vi "Load Waveform From TDMS.vi"(0 "TDMS File Path":path, 5 "Waveform Name (File Name)":string, 11 "error in (no error)":errorcluster) -> (4 "Waveform":T1={"Waveform Name"="Wfm", "Waveform"={"x0"=0.0, "dx"=0.0, "y"=[]}, "Signal Bandwidth (Hz)"=0.0, "PAPR (dB)"=0.0, "Burst Length (s)"=0.0, "Sample Rate"=0.0, "Burst Start Locations"=[], "Burst Stop Locations"=[], "Idle Duration Present?"=FALSE, "Runtime Scaling"=0.0} {"Runtime Scaling" format="%#_6p"; "Sample Rate" format="%#_6p"; "Burst Length (s)" format="%#_6p"; "PAPR (dB)" format="%.2f"; "Signal Bandwidth (Hz)" format="%.2f"; "Waveform"."y" format="%.2f"; "Waveform"."dx" format="%^.2e"; "Waveform"."x0" format="%^.2e"}, 15 "error out":errorcluster)   [LabVIEW 2016, in "SG.lvlib"]
uses:
  SG.lvlib
  Typedefs/Waveform.ctl
  <instrlib>/niRFSGPlayback/niRFSGPlayback Read Waveform From File (1 Wfm,TDMS, CSG).vi
  Utilities/RDLUtilities.lvlib
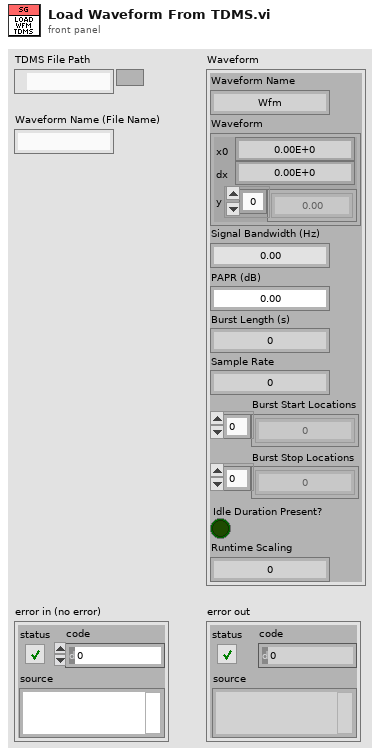
[diagram p1: front panel]
types:
  T1 = typedef "SG.lvlib/Waveform.ctl" = cluster{"Waveform Name":string, "Waveform":cluster{"x0":dbl, "dx":dbl, "y":csg[]}, "Signal Bandwidth (Hz)":dbl, "PAPR (dB)":dbl, "Burst Length (s)":dbl, "Sample Rate":dbl, "Burst Start Locations":i32[], "Burst Stop Locations":i32[], "Idle Duration Present?":bool, "Runtime Scaling":dbl}
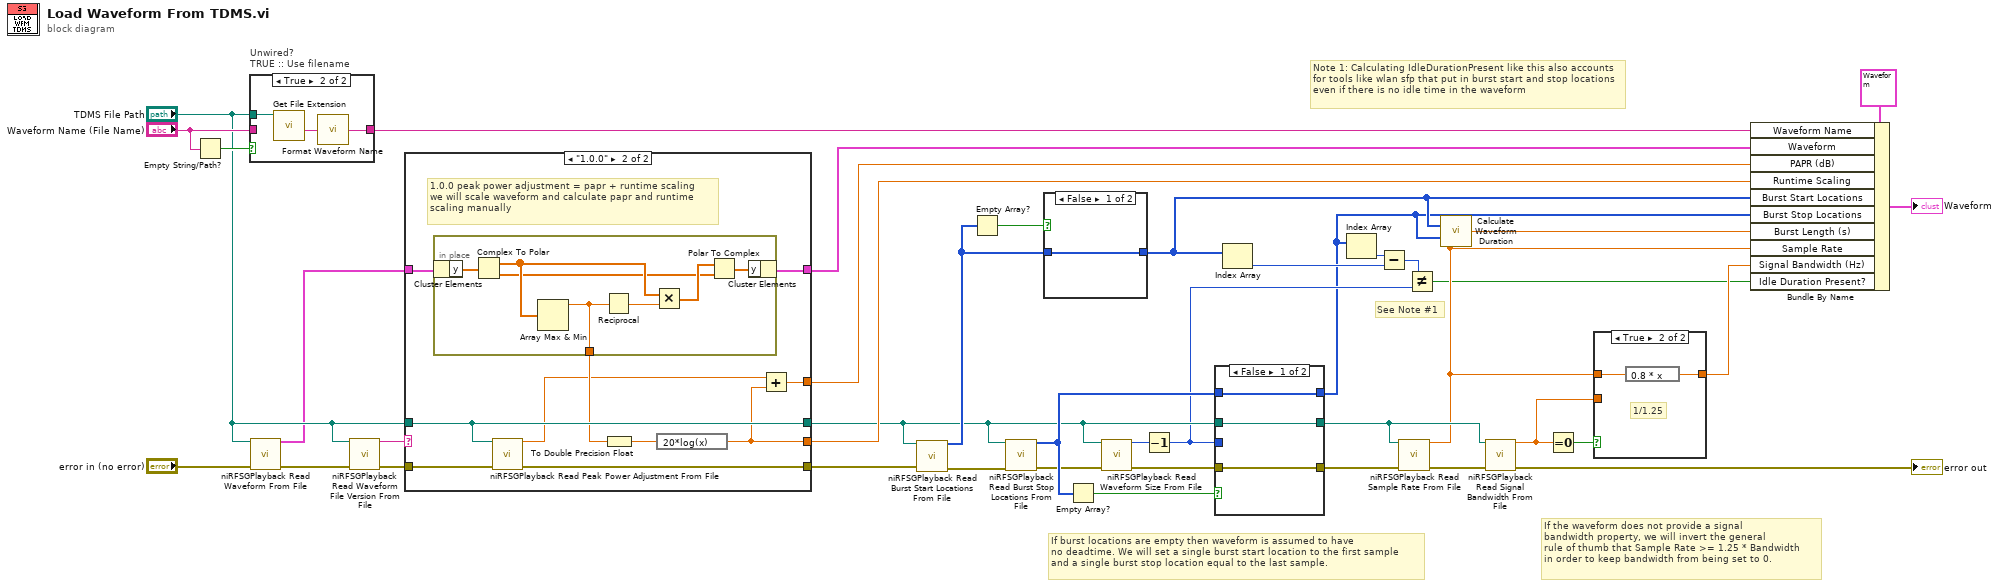
[diagram p0: block diagram]
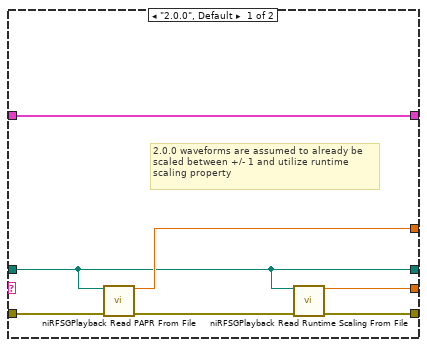
[diagram p2: hidden frame]
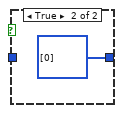
[diagram p4: hidden frame]
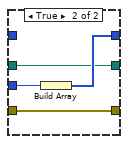
[diagram p5: hidden frame]
diagram:
  # "See Note #1"
  # "Note 1: Calculating IdleDurationPresent like this also accounts for tools like wlan sfp that put in burst start and stop locations even if there is no idle time in the waveform"
  # "If the waveform does not provide a signal\nbandwidth property, we will invert the general\nrule of thumb that Sample Rate >= 1.25 * Bandwidth\nin order to keep bandwidth from being set to 0."
  # "If burst locations are empty then waveform is assumed to have\nno deadtime. We will set a single burst start location to the first sample \nand a single burst stop location equal to the last sample."
  n1 = Empty String/Path?(string/path="Waveform Name (File Name)") -> (empty?=w34:bool)
  n2 = case "Unwired?\nTRUE :: Use filename" shown="True" w34 {
    tunnel: [w41 w42] -> w32
    tunnel: "Waveform Name (File Name)" -> [w41 _]
    tunnel: "TDMS File Path" -> [_ w44]
    frame False {
    }
    frame True {
      n3 = call <vilib>:"Get File Extension.vi"("file"=w44) -> ("filename without extension"=w43:string)  [unwired: 6 in, 4 out]
      n4 = call "Format Waveform Name.vi"("Waveform File Name"=w43) -> ("Waveform Name"=w42:string)
    }
  }
  n5 = call-poly <instrlib>:"niRFSGPlayback Read Waveform From File.vi"("file path"="TDMS File Path", "error in"="error in (no error)") -> ("waveform"=w20:cluster{"t0":dbl, "dt":dbl, "y":csg[]}, "error out"=w39:errorcluster)  [unwired: 12 in]
  n6 = call <instrlib>:"niRFSGPlayback Read Waveform File Version From File.vi"("file path"="TDMS File Path", "error in"=w39) -> ("waveform file version"=w38:string, "error out"=w37:errorcluster)  [unwired: 12 in]
  n7 = case shown="\"1.0.0\"" w38 {
    tunnel: w37 -> [w50 w61]
    tunnel: [w47 w59] -> w6
    tunnel: [w51 w52] -> w36
    tunnel: [w48 w60] -> w35
    tunnel: "TDMS File Path" -> [w47 w59]
    tunnel: [w46 w53] -> w21
    tunnel: w20 -> [w45 w58]
    tunnel: [w45 w57] -> w19
    frame "2.0.0", Default {
      # "2.0.0 waveforms are assumed to already be\nscaled between +/- 1 and utilize runtime\nscaling property"
      n8 = call <instrlib>:"niRFSGPlayback Read PAPR From File.vi"("file path"=w47, "error in"=w50) -> ("PAPR"=w51:dbl, "error out"=w49:errorcluster)  [unwired: 12 in]
      n9 = call <instrlib>:"niRFSGPlayback Read Runtime Scaling From File.vi"("file path"=w47, "error in"=w49) -> ("runtime scaling"=w46:dbl, "error out"=w48:errorcluster)  [unwired: 12 in]
    }
    frame "1.0.0" {
      # "1.0.0 peak power adjustment = papr + runtime scaling\nwe will scale waveform and calculate papr and runtime\nscaling manually"
      n10 = in-place {
        in-place-border: [w64] -> w56
        n11 = in-place-cluster #1(w58) -> ("y"=w63:csg[])
        n12 = Complex To Polar(r * e^(i*theta)=w63) -> (r=w67:sgl[], theta=w66:sgl[])
        n13 = Array Max & Min(array=w67) -> (max value=w64:sgl)  [unwired: 3 out]
        n14 = Reciprocal(x=w64) -> (1/x=w62:sgl)
        n15 = Multiply(x=w67, y=w62) -> (x*y=w68:sgl[])
        n16 = Polar To Complex(1:w66, 2:w68) -> (0:w65:csg[])
        n17 = in-place-cluster #1("y"=w65) -> (w57:cluster{"t0":dbl, "dt":dbl, "y":csg[]})
      }
      n18 = call <instrlib>:"niRFSGPlayback Read Peak Power Adjustment From File.vi"("file path"=w59, "error in"=w61) -> ("peak power adjustment"=w54:dbl, "error out"=w60:errorcluster)  [unwired: 12 in]
      n19 = To Double Precision Float(number=w56) -> (double precision float=w55:dbl)
      n20 = expression code="20*log(x)"(w55) -> (w53:dbl)
      n21 = Add(x=w54, y=w53) -> (x+y=w52:dbl)
    }
  }
  n22 = call <instrlib>:"niRFSGPlayback Read Burst Start Locations From File.vi"("file path"=w6, "error in"=w35) -> ("burst start locations"=w26:i32[], "error out"=w30:errorcluster)  [unwired: 12 in]
  n23 = Empty Array?(array=w26) -> (empty?=w27:bool)
  n24 = call <instrlib>:"niRFSGPlayback Read Burst Stop Locations From File.vi"("file path"=w6, "error in"=w30) -> ("burst stop locations"=w23:i32[], "error out"=w8:errorcluster)  [unwired: 12 in]
  n25 = case shown="False" w27 {
    tunnel: w26 -> [w69 _]
    tunnel: [w69 i32[] [0]] -> w11
    frame False {
    }
    frame True {
    }
  }
  n26 = Empty Array?(array=w23) -> (empty?=w24:bool)
  n27 = call <instrlib>:"niRFSGPlayback Read Waveform Size From File.vi"("file path"=w6, "error in"=w8) -> ("waveform size"=w5:i32, "error out"=w7:errorcluster)  [unwired: 12 in]
  n28 = Decrement(x=w5) -> (x-1=w4:i32)
  n29 = case shown="False" w24 {
    tunnel: w6 -> [w71 w76]
    tunnel: w7 -> [w72 w74]
    tunnel: [w72 w74] -> w25
    tunnel: w23 -> [w73 _]
    tunnel: [w73 w77] -> w2
    tunnel: [w71 w76] -> w22
    tunnel: w4 -> [_ w75]
    frame False {
    }
    frame True {
      n30 = Build Array(w75) -> (w77:i32[])
    }
  }
  n31 = Index Array(array=w11) -> (element=w10:i32)  [unwired: 1 in]
  n32 = Index Array(array=w2) -> (element=w9:i32)  [unwired: 1 in]
  n33 = Subtract(x=w9, y=w10) -> (x-y=w1:i32)
  n34 = call <instrlib>:"niRFSGPlayback Read Sample Rate From File.vi"("file path"=w22, "error in"=w25) -> ("sample rate"=w12:dbl, "error out"=w28:errorcluster)  [unwired: 12 in]
  n35 = Not Equal?(x=w1, y=w4) -> (x != y?=w3:bool)
  n36 = call "Calculate Waveform Duration.vi"("Sample Rate"=w12, "Burst Start Locations"=w11, "Burst Stop Locations"=w2) -> ("Burst Length (s)"=w13:dbl)  [unwired: 12 in]
  n37 = call <instrlib>:"niRFSGPlayback Read Signal Bandwidth From File.vi"("file path"=w22, "error in"=w28) -> ("signal bandwidth"=w16:dbl, "error out"=→"error out":errorcluster)  [unwired: 12 in]
  n38 = Equal To 0?(x=w16) -> (x = 0?=w17:bool)
  n39 = case shown="True" w17 {
    tunnel: w12 -> [_ w80]
    tunnel: w16 -> [w78 _]
    tunnel: [w78 w79] -> w15
    frame False {
    }
    frame True {
      # "1/1.25"
      n40 = expression code="0.8 * x"(w80) -> (w79:dbl)
    }
  }
  n41 = Bundle By Name(cluster=T1 {"Waveform Name"="Wfm", "Waveform"={"x0"=0.0, "dx"=0.0, "y"=[]}, "Signal Bandwidth (Hz)"=0.0, "PAPR (dB)"=0.0, "Burst Length (s)"=0.0, "Sample Rate"=0.0, "Burst Start Locations"=[], "Burst Stop Locations"=[], "Idle Duration Present?"=FALSE, "Runtime Scaling"=0.0} ("Waveform"), "Waveform Name"=w32, "Waveform"=w19, "PAPR (dB)"=w36, "Runtime Scaling"=w21, "Burst Start Locations"=w11, "Burst Stop Locations"=w2, "Burst Length (s)"=w13, "Sample Rate"=w12, "Signal Bandwidth (Hz)"=w15, "Idle Duration Present?"=w3) -> (→"Waveform":T1)
